vi "robotkontrolkoordinat.vi"() -> ()   [LabVIEW 2016]
panel:
  out "Q1":dbl
  out "Q2":dbl
  in  "l2":dbl
  in  "l1":dbl
  in  "y":dbl
  in  "x":dbl
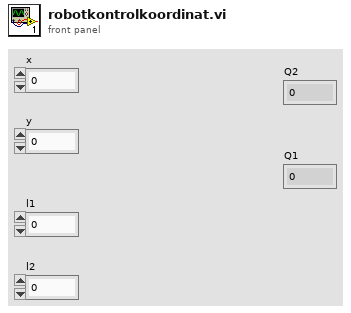
[diagram p1: front panel]
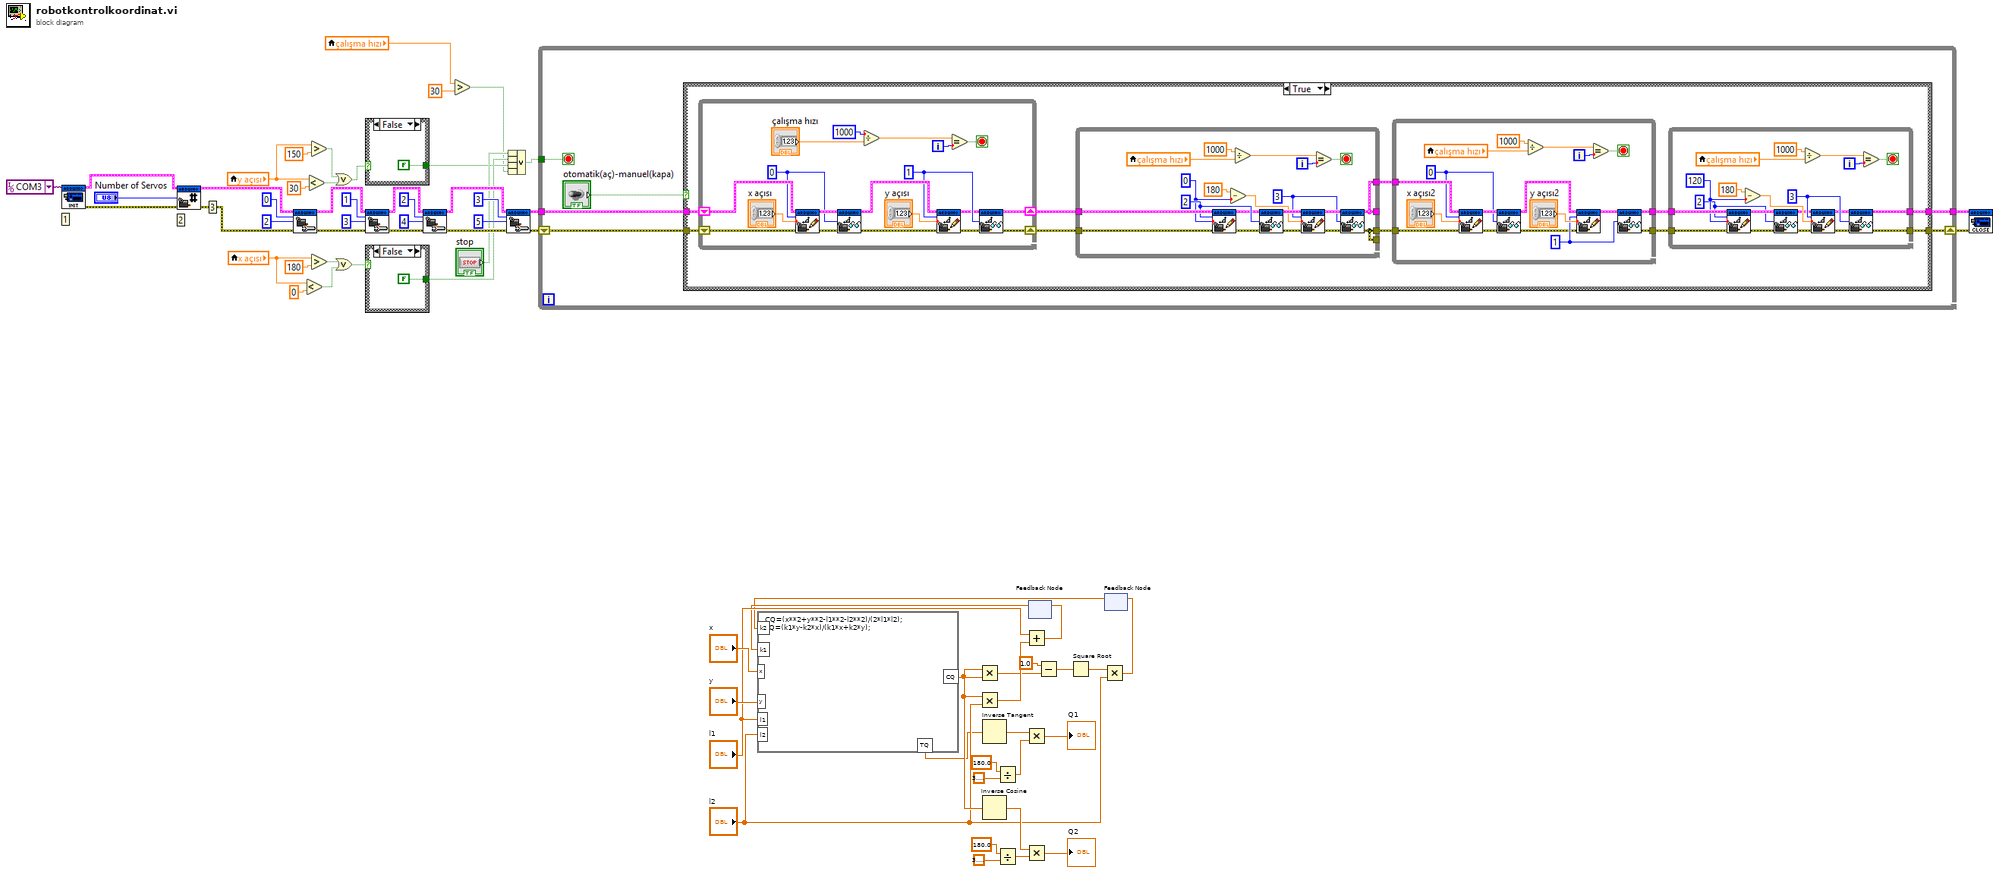
[diagram p0: block diagram]
diagram:
  n1 = Divide(x=180.0, y=3.141592653589793) -> (x/y=w2:dbl)
  n2 = Divide(x=180.0, y=3.141592653589793) -> (x/y=w20:dbl)
  n3 = feedback #1() -> (w9:dbl)  [unwired: 1 in]
  n4 = feedback #2() -> (w7:dbl)  [unwired: 1 in]
  n5 = formula code="CQ=(x**2+y**2-l1**2-l2**2)/(2*l1*l2);\nTQ=(k1*y-k2*x)/(k1*x+k2*y);"("x"="x", "y"="y", "l1"="l1", "l2"="l2", "k1"=w9, "k2"=w7) -> ("CQ"=w16:dbl, "TQ"=w6:dbl)
  n6 = Multiply(x=w16, y=w16) -> (x*y=w14:dbl)
  n7 = Multiply(x=w16, y="l2") -> (x*y=w19:dbl)
  n8 = Inverse Tangent(1:w6) -> (0:w5:dbl)
  n9 = Inverse Cosine(1:w16) -> (0:w21:dbl)
  n10 = Add(x="l1", y=w19) -> (x+y=w10:dbl)
  n11 = Multiply(x=w5, y=w2) -> (x*y=→"Q1":dbl)
  n12 = Multiply(x=w21, y=w20) -> (x*y=→"Q2":dbl)
  n13 = feedback-in #1(w10) -> ()
  n14 = Subtract(x=1.0, y=w14) -> (x-y=w13:dbl)
  n15 = Square Root(x=w13) -> (sqrt(x)=w12:dbl)
  n16 = Multiply(x=w12, y="l2") -> (x*y=w8:dbl)
  n17 = feedback-in #2(w8) -> ()
